vi "Populate Communication Specific Objects.vi"(8 "error in":errorcluster, 10 "EDS":refnum<class "Electronic Datasheet.lvclass">, 11 "object in":refnum<class "Object Dictionary UI.lvclass">) -> (0 "error out":errorcluster, 3 "object out":refnum<class "Object Dictionary UI.lvclass">)   [LabVIEW 2024, in "Object Dictionary UI.lvlib" / "Object Dictionary UI.lvclass"]
uses:
  Object Dictionary UI.lvclass
  Object Dictionary UI.lvclass/Object Dictionary UI.ctl
  EDS-File-Viewer/Electronic Datasheet/Electronic Datasheet.lvclass
  EDS-File-Viewer/Core/OD Entry/OD Entry.lvclass
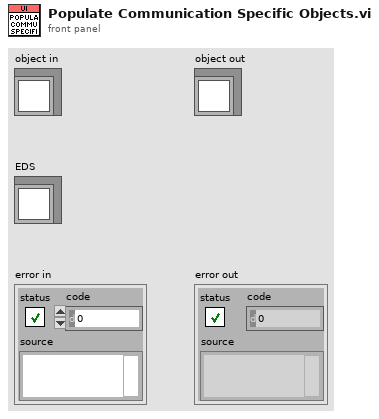
[diagram p1: front panel]
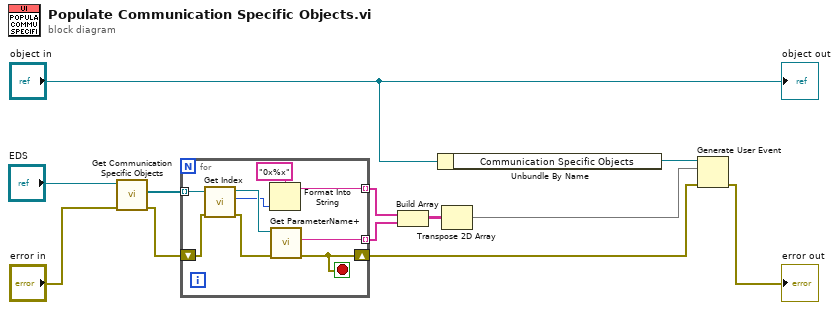
[diagram p0: block diagram]
diagram:
  n1 = call "Get Communication Specific Objects.vi"("error in"="error in", "Electronic Datasheet"="EDS") -> ("error out"=w7:errorcluster, "Entries"=w8:refnum<class "OD Entry.lvclass">[])  [unwired: 7 in, 1 out]
  n2 = for {
    tunnel: w8 -> [w21] mode=indexing
    tunnel: [w18] -> w3 mode=indexing
    shift-right: [w13] -> w2
    shift-left: w7 -> [w17]
    tunnel: [w14] -> w4 mode=indexing
    stop <- w13 stop-if-true
    n3 = call "Get Index.vi"("Error In"=w17, "reference in"=w21) -> ("Error Out"=w19:errorcluster, "Index"=w16:u16, "reference out"=w20:refnum<class "OD Entry.lvclass">)  [unwired: 7 in]
    n4 = Format Into String(format string="0x%x", w16) -> (resulting string=w14:string)  [unwired: 2 in, 1 out]
    n5 = call "Get ParameterName+.vi"("Error In"=w19, "reference in"=w20) -> ("Error Out"=w13:errorcluster, "ParameterName"=w18:string)  [unwired: 6 in, 2 out]
  }
  n6 = Build Array(w4, w3) -> (w5:string[][])
  n7 = Unbundle By Name("object in") -> ("Communication Specific Objects"=w6:refnum<user-event>)
  n8 = Transpose 2D Array(2D array=w5) -> (transposed array=w1:string[][])
  n9 = Generate User Event(user event=w6, event data cluster=w1, error in=w2) -> (error out=→"error out":errorcluster)  [unwired: 1 in, 1 out]
  "object out" <- "object in"
